vi "binaryStringToInteger.vi"(1 "Binary String":string) -> (0 "Integer Output":i32)   [LabVIEW 2017]
doc: "Converts a string of four bytes to an integer."
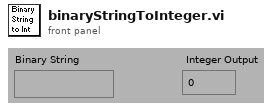
[diagram p1: front panel]
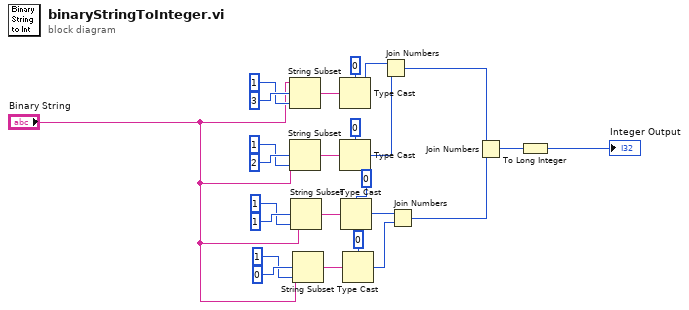
[diagram p0: block diagram]
diagram:
  n1 = String Subset(string="Binary String", offset (0)=3, length (rest)=1 ("length")) -> (substring=w19:string)
  n2 = String Subset(string="Binary String", offset (0)=2, length (rest)=1 ("length")) -> (substring=w23:string)
  n3 = String Subset(string="Binary String", offset (0)=1, length (rest)=1 ("length")) -> (substring=w11:string)
  n4 = String Subset(string="Binary String", offset (0)=0, length (rest)=1 ("length")) -> (substring=w15:string)
  n5 = Type Cast(type=u8 0, x=w19) -> (*(type *) &x=w9:u8)
  n6 = Type Cast(type=u8 0, x=w23) -> (*(type *) &x=w8:u8)
  n7 = Type Cast(type=u8 0, x=w11) -> (*(type *) &x=w7:u8)
  n8 = Type Cast(type=u8 0, x=w15) -> (*(type *) &x=w6:u8)
  n9 = Join Numbers(hi=w9, lo=w8) -> ((hi.lo)=w4:u16)
  n10 = Join Numbers(hi=w7, lo=w6) -> ((hi.lo)=w5:u16)
  n11 = Join Numbers(hi=w4, lo=w5) -> ((hi.lo)=w3:u32)
  n12 = To Long Integer(number=w3) -> (32bit integer=→"Integer Output":i32)
